vi "Get Item Property List.vi"(8 "error in (no error)":errorcluster, 11 "Item Reference in":T1 format="%.0x") -> (0 "error out":errorcluster, 1 "Values":variant[](array[variant]), 2 "Property Names":string[](array[string]), 3 "Item Reference out":T1 format="%.0x")   [LabVIEW 2013, in "Hierarchy Framework.lvlib" / "Item.lvclass"]
doc: "Returns all the <B>Property Names</B> and <B>Values</B> of the properties associated with a custom device item."
uses:
  Item.lvclass
  Ctls/Item Reference.ctl
  Generic/Generic.lvclass
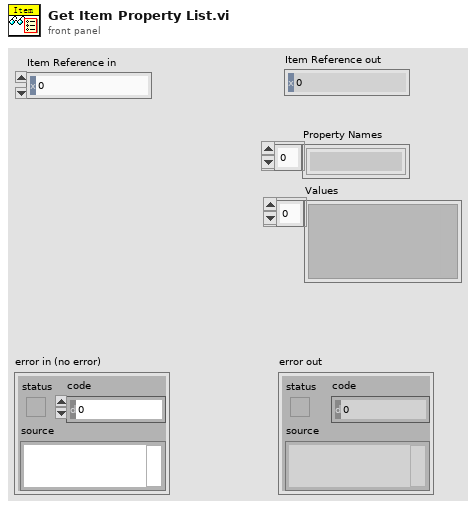
[diagram p1: front panel]
types:
  T1 = typedef "Hierarchy Framework.lvlib/Item.lvclass/Item Reference.ctl" = u64
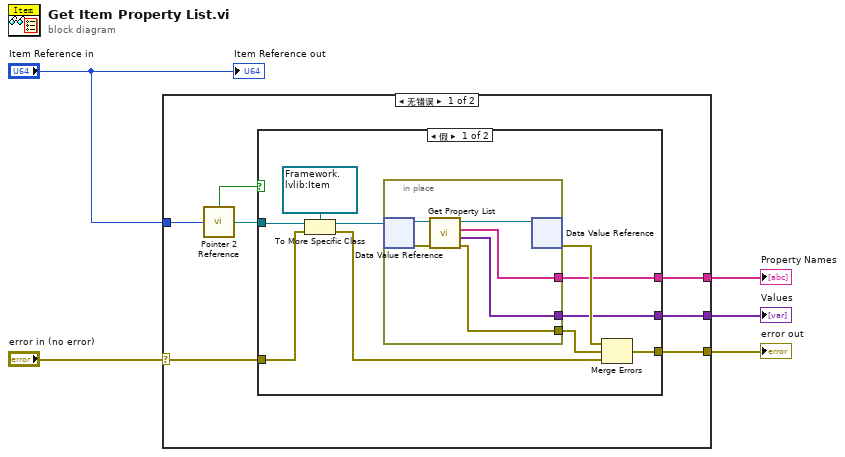
[diagram p0: block diagram]
diagram:
  n1 = case shown="无错误" "error in (no error)" {
    selector: "error in (no error)" -> [w11 w30]
    tunnel: "Item Reference in" -> [w8 _]
    tunnel: [w12 w30] -> w4
    tunnel: [w10 _] -> w2
    tunnel: [w9 _] -> w1
    frame No Error {
      n2 = call "Pointer 2 Reference.vi"("Pointer"=w8) -> ("Not A Refnum?"=w7:bool, "Generic Reference"=w6:refnum<data-value>)
      n3 = case shown="假" w7 {
        tunnel: w11 -> [w16 w29]
        tunnel: [w21 w29] -> w12
        tunnel: [w20 _] -> w10
        tunnel: [w19 _] -> w9
        tunnel: w6 -> [w17 _]
        frame False {
          n4 = To More Specific Class(target class=refnum<data-value> refnum ("Item"), reference=w17, error in=w16) -> (specific class reference=w13:refnum<data-value>, error out=w15:errorcluster)
          n5 = in-place {
            in-place-border: [w25] -> w20
            in-place-border: [w24] -> w19
            in-place-border: [w23] -> w18
            n6 = in-place-dvr #1(w13) -> (w28:refnum<class "Item.lvclass">, w26:errorcluster)
            n7 = call-dynamic "Get Property List.vi"("error in (no error)"=w26, "Item输入"=w28) -> ("error out"=w23:errorcluster, "Values"=w24:variant[], "Property Names"=w25:string[], "Item输出"=w27:refnum<class "Item.lvclass">)  [unwired: 6 in]
            n8 = in-place-dvr #1(w27) -> (w22:errorcluster)  [unwired: 1 out]
          }
          n9 = Merge Errors(w22, w18, w15) -> (w21:errorcluster)
        }
        frame True {
        }
      }
    }
    frame Error {
    }
  }
  "error out" <- w4
  "Property Names" <- w2
  "Values" <- w1
  "Item Reference out" <- "Item Reference in"
